vi "Get Status.vi"(11 "error in (no error)":errorcluster) -> (4 "Status":T1=enum."Alarm", 6 "Limit switch":cluster{"X":bool, "Y":bool, "Z":bool}, 8 "Current position":cluster{"X":sgl, "Y":sgl, "Z":sgl}, 10 "Status information":string, 15 "error out":errorcluster)   [LabVIEW 2024, in "GRBL 1.1.lvlib"]
doc: "Get the status of the GRBL controller"
uses:
  GRBL 1.1.lvlib
  Status.ctl
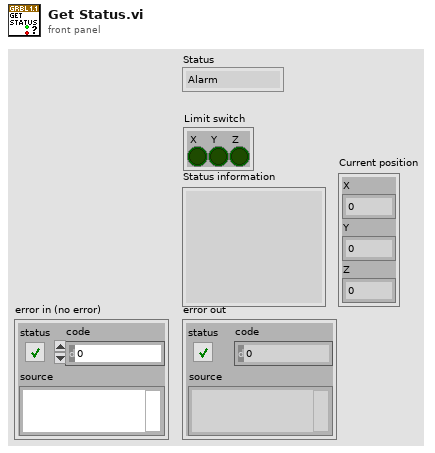
[diagram p1: front panel]
types:
  T1 = typedef "GRBL 1.1.lvlib/Status.ctl" = enum16{"", "Alarm", "Idle", "Run", "Home"}
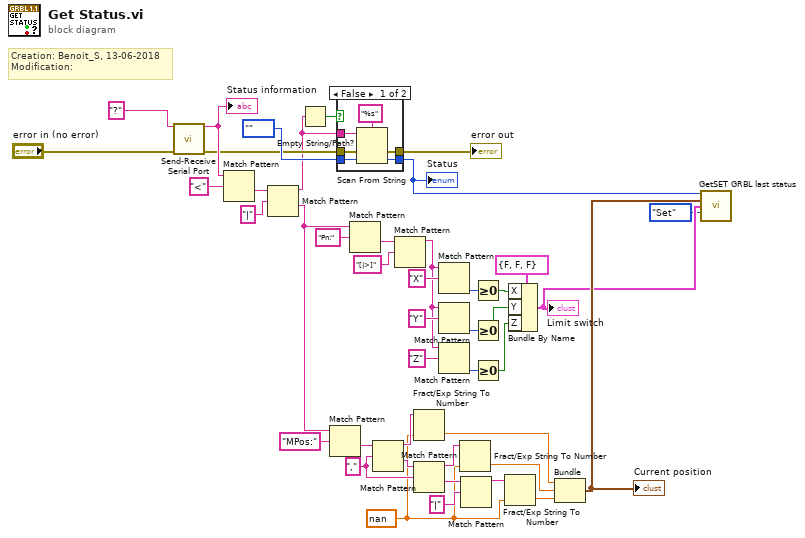
[diagram p0: block diagram]
diagram:
  w9 = sgl nan ("default (0 DBL)")
  w13 = "," ("regular expression")
  # "Creation: Benoit_S, 13-06-2018\nModification:"
  n1 = call "Send-Receive Serial Port.vi"("Data to write"="?", "error in (no error)"="error in (no error)") -> ("Data read"=w28:string, "error out"=w23:errorcluster)  [unwired: 12 in]
  "Status information" <- w28
  n2 = Match Pattern(string=w28, regular expression="<") -> (after substring=w26:string)  [unwired: 1 in, 3 out]
  n3 = Match Pattern(string=w26, regular expression="|") -> (before substring=w22:string, after substring=w19:string)  [unwired: 1 in, 2 out]
  n4 = Empty String/Path?(string/path=w22) -> (empty?=w21:bool)
  n5 = Match Pattern(string=w19, regular expression="MPos:") -> (after substring=w17:string)  [unwired: 1 in, 3 out]
  n6 = case shown="False" w21 {
    tunnel: Status."" ("Status") -> [w49 w51]
    tunnel: [w48 w51] -> w5
    tunnel: w22 -> [w46 _]
    tunnel: w23 -> [w45 w50]
    tunnel: [w44 w50] -> w20
    frame False {
      n7 = Scan From String(format string="%s", input string=w46, error in=w45, default 1=w49) -> (error out=w44:errorcluster, output 1=w48:T1)  [unwired: 1 in, 2 out]
    }
    frame True {
    }
  }
  "error out" <- w20
  "Status" <- w5
  n8 = Match Pattern(string=w19, regular expression="Pn:") -> (after substring=w41:string)  [unwired: 1 in, 3 out]
  n9 = Match Pattern(string=w17, regular expression=w13) -> (before substring=w12:string, after substring=w16:string)  [unwired: 1 in, 2 out]
  n10 = Match Pattern(string=w41, regular expression="[|>]") -> (before substring=w29:string)  [unwired: 1 in, 3 out]
  n11 = Fract/Exp String To Number(string=w12, default (0 dbl)=w9) -> (number=w8:sgl)  [unwired: 2 in, 1 out]
  n12 = Match Pattern(string=w16, regular expression=w13) -> (before substring=w11:string, after substring=w15:string)  [unwired: 1 in, 2 out]
  n13 = Match Pattern(string=w29, regular expression="X") -> (offset past match=w36:i32)  [unwired: 1 in, 3 out]
  n14 = Match Pattern(string=w29, regular expression="Y") -> (offset past match=w35:i32)  [unwired: 1 in, 3 out]
  n15 = Match Pattern(string=w29, regular expression="Z") -> (offset past match=w34:i32)  [unwired: 1 in, 3 out]
  n16 = Fract/Exp String To Number(string=w11, default (0 dbl)=w9) -> (number=w7:sgl)  [unwired: 2 in, 1 out]
  n17 = Match Pattern(string=w15, regular expression="|") -> (before substring=w10:string)  [unwired: 1 in, 3 out]
  n18 = Greater Or Equal To 0?(x=w36) -> (x >= 0?=w30:bool)
  n19 = Greater Or Equal To 0?(x=w35) -> (x >= 0?=w31:bool)
  n20 = Greater Or Equal To 0?(x=w34) -> (x >= 0?=w32:bool)
  n21 = Fract/Exp String To Number(string=w10, default (0 dbl)=w9) -> (number=w6:sgl)  [unwired: 2 in, 1 out]
  n22 = Bundle By Name(cluster=cluster{"X":bool, "Y":bool, "Z":bool} {"X"=FALSE, "Y"=FALSE, "Z"=FALSE} ("Limit switch"), "X"=w30, "Y"=w31, "Z"=w32) -> (w3:cluster{"X":bool, "Y":bool, "Z":bool})
  "Limit switch" <- w3
  n23 = Bundle(w8, w7, w6) -> (w4:cluster{sgl, sgl, sgl})  [unwired: 1 in]
  "Current position" <- w4
  n24 = call "GetSET GRBL last status.vi"("Status in"=w5, "Current position in"=w4, "Limit switch in"=w3, "Get/Set"=enum16{"Get", "Set"}."Set") -> ()  [unwired: 8 in, 4 out]
